vi "Remcon32 command.vi"(5 "Close session":bool, 7 "Initialization":bool, 8 "error in":errorcluster, 10 "SEM command":string, 11 "COM port in":refnum<visa-resource-name>) -> (0 "error out":errorcluster, 1 "return count":u32, 2 "SEM reply":string, 3 "COM port out":refnum<visa-resource-name>)   [LabVIEW 2018]
uses:
  <vilib>/Instr/_visa.llb/VISA Configure Serial Port (Instr).vi
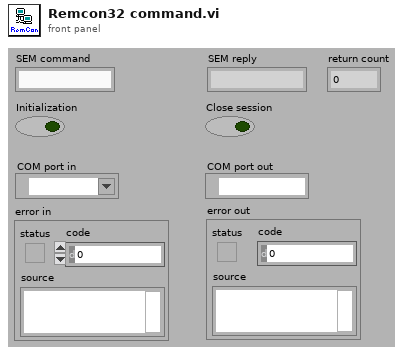
[diagram p1: front panel]
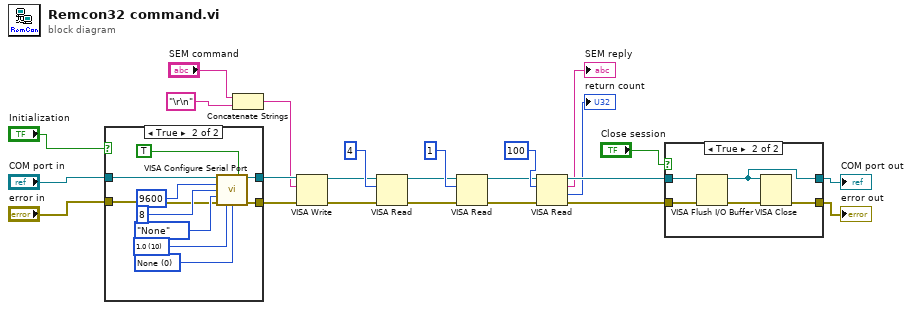
[diagram p0: block diagram]
diagram:
  n1 = case shown="True" "Initialization" {
    tunnel: [w26 w30] -> w17
    tunnel: [w25 w29] -> w16
    tunnel: "COM port in" -> [w26 w28]
    tunnel: "error in" -> [w25 w27]
    frame False {
    }
    frame True {
      w35 = u16 0 items=["None", "XON/XOFF", "RTS/CTS", "XON/XOFF & RTS/CTS", "DTR/DSR", "XON/XOFF & DTR/DSR"] ("flow control (0:none)")
      w34 = u16 10 items=["1.0"=10, "1.5"=15, "2.0"=20] ("stop bits (10: 1 bit)")
      n2 = call-poly "VISA Configure Serial Port"("VISA resource name"=w28, "Enable Termination\nChar (T)"=TRUE ("Enable Termination\nChar (T)"), "baud rate (9600)"=u32 9600, "data bits (8)"=u16 8, "parity (0:none)"=enum16{"None", "Odd", "Even", "Mark", "Space"}."None", "error in (no error)"=w27, "stop bits (10: 1 bit)"=w34, "flow control (0:none)"=w35) -> ("VISA resource name out"=w30:refnum<visa-resource-name>, "error out"=w29:errorcluster)  [unwired: 6 out]
    }
  }
  n3 = Concatenate Strings("SEM command", "\r\n" ("write buffer")) -> (w10:string)
  n4 = VISA Write(VISA resource name=w17, write buffer=w10, error in (no error)=w16) -> (VISA resource name out=w22:refnum<visa-resource-name>, error out=w21:errorcluster)  [unwired: 1 out]
  n5 = VISA Read(VISA resource name=w22, byte count=u32 4, error in (no error)=w21) -> (VISA resource name out=w1:refnum<visa-resource-name>, error out=w4:errorcluster)  [unwired: 2 out]
  n6 = VISA Read(VISA resource name=w1, byte count=u32 1, error in (no error)=w4) -> (VISA resource name out=w2:refnum<visa-resource-name>, error out=w3:errorcluster)  [unwired: 2 out]
  n7 = VISA Read(VISA resource name=w2, byte count=u32 100, error in (no error)=w3) -> (VISA resource name out=w12:refnum<visa-resource-name>, read buffer=→"SEM reply":string, return count=→"return count":u32, error out=w11:errorcluster)
  n8 = case shown="True" "Close session" {
    tunnel: w12 -> [w38 w42]
    tunnel: w11 -> [w37 w41]
    tunnel: [w38 w40] -> w14
    tunnel: [w37 w43] -> w13
    frame False {
    }
    frame True {
      n9 = VISA Flush I/O Buffer(VISA resource name=w42, error in (no error)=w41) -> (VISA resource name out=w40:refnum<visa-resource-name>, error out=w39:errorcluster)  [unwired: 1 in]
      n10 = VISA Close(VISA resource name=w40, error in (no error)=w39) -> (error out=w43:errorcluster)
    }
  }
  "COM port out" <- w14
  "error out" <- w13
